vi "AFT Update Coefficients (Real, PtByPt).vi"(6 "step size":dbl=-1.0, 8 "error in (no error)":errorcluster, 10 "e(n)":dbl, 11 "adaptive filter in":refnum<k20>) -> (0 "error out":errorcluster, 3 "adaptive filter out":refnum<k20>)   [LabVIEW 2017, in "NI_AdaptiveFilter.lvlib"]
doc: "Updates the coefficients of an adaptive filter point by point. Use this VI with the AFT Filter Signal VI to update the coefficients of an adaptive filter. You must use the least mean squares (LMS) or recursive least squares (RLS) algorithms to create the adaptive filter. Wire data to the <B>e(n)</B> input to determine the polymorphic instance to use or manually select the instance. The data type of the adaptive filter that you wire to the <B>adaptive filter in</B> input must match the instance of the AFT Update Coefficients VI."
uses:
  <vilib>/addons/Adaptive Filters/NI_AdaptiveFilter.lvlib
  <resource>/AdaptiveFilters.dll
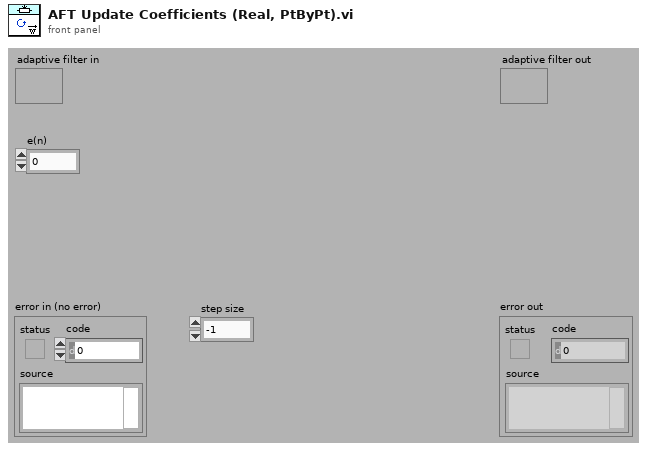
[diagram p1: front panel]
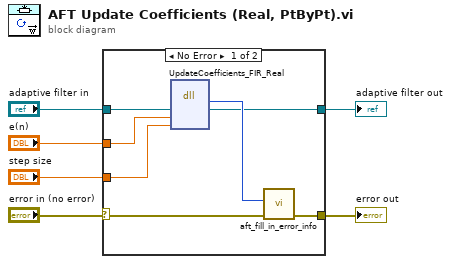
[diagram p0: block diagram]
diagram:
  n1 = case shown="No Error" "error in (no error)" {
    selector: "error in (no error)" -> [w12 w15]
    tunnel: [w10 w15] -> w6
    tunnel: "adaptive filter in" -> [w8 w14]
    tunnel: "e(n)" -> [w13 _]
    tunnel: [w7 w14] -> w2
    tunnel: "step size" -> [w9 _]
    frame No Error {
      n2 = dll-call lib="C:/Program Files/National Instruments/LabVIEW 2017/resource/AdaptiveFilters.dll" fn="UpdateCoefficients_FIR_Real" ("Complex Data Initialization")("pSession"=w8, "e"=w13, "mu"=w9) -> ("err"=w11:i32, "pSession"=w7:refnum<k20>)  [unwired: 5 in, 2 out]
      n3 = call <vilib>:"aft_fill_in_error_info.vi"("error in"=w12, "status code"=w11) -> ("error out"=w10:errorcluster)  [unwired: 2 in, 7 out]
    }
    frame Error {
    }
  }
  "error out" <- w6
  "adaptive filter out" <- w2
